vi "LineDraw.vi"(6 "Array":dbl[][](array[numeric]), 8 "Point Y":dbl, 9 "Point X":dbl, 10 "Vehicle Pos Y":dbl, 11 "Vehicle Pos X":dbl) -> (2 "Array 2":dbl[][](array[numeric]))   [LabVIEW 2017]
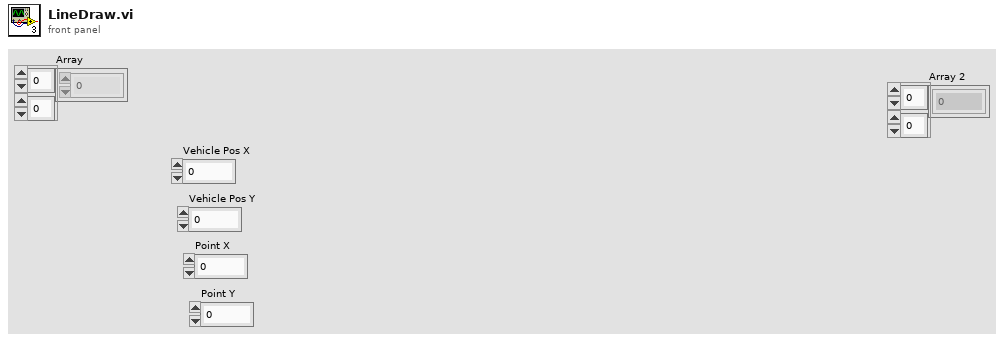
[diagram p1: front panel]
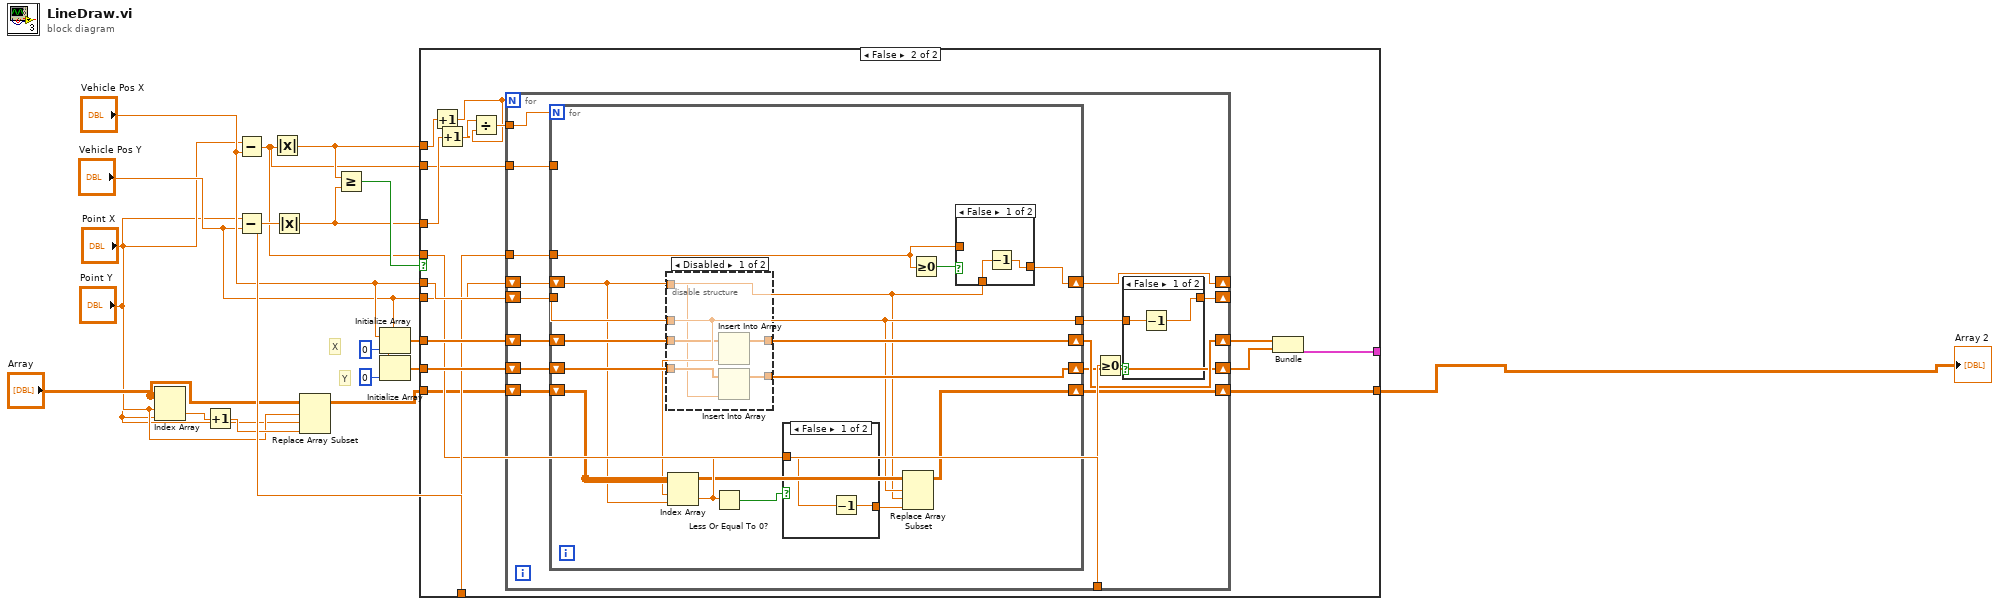
[diagram p0: block diagram]
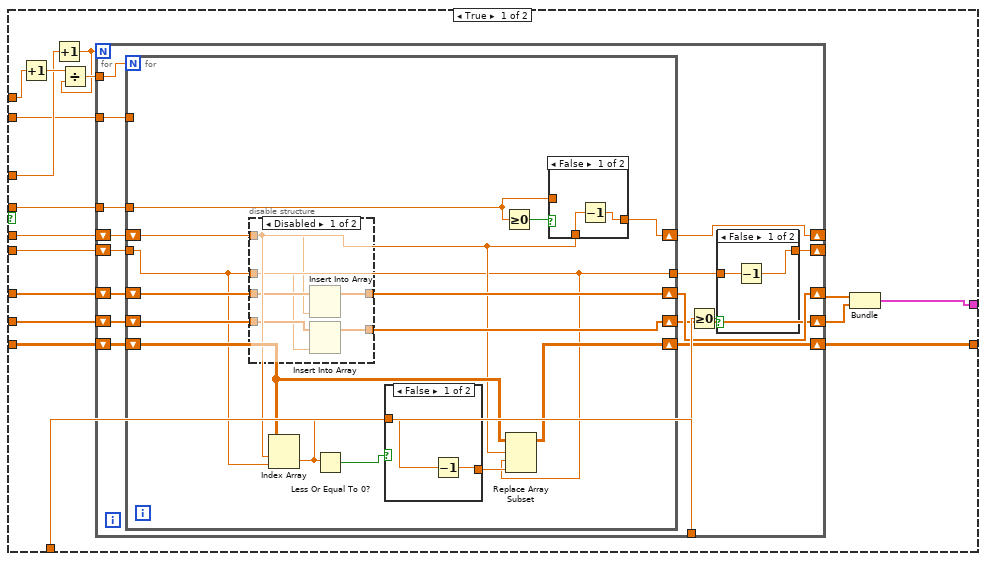
[diagram p2: hidden frame]
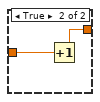
[diagram p3: hidden frame]
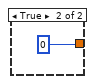
[diagram p5: hidden frame]
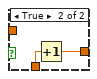
[diagram p6: hidden frame]
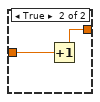
[diagram p7: hidden frame]
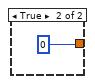
[diagram p9: hidden frame]
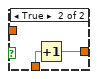
[diagram p10: hidden frame]
diagram:
  # "Y"
  # "X"
  n1 = Index Array(array="Array", index (row)="Point X", index (col)="Point Y") -> (element=w4:dbl)
  n2 = Increment(x=w4) -> (x+1=w3:dbl)
  n3 = Subtract(x="Point X", y="Vehicle Pos X") -> (x-y=w14:dbl)
  n4 = Subtract(x="Point Y", y="Vehicle Pos Y") -> (x-y=w15:dbl)
  n5 = Absolute Value(x=w14) -> (abs(x)=w16:dbl)
  n6 = Absolute Value(x=w15) -> (abs(x)=w17:dbl)
  n7 = Replace Array Subset(array="Array", new element=w3, index (row)="Point X", index (col)="Point Y") -> (w5:dbl[][])
  n8 = Greater Or Equal?(x=w16, y=w17) -> (x >= y?=w18:bool)
  n9 = Initialize Array("Vehicle Pos X", 0 ("dimension size")) -> (w11:dbl[])
  n10 = Initialize Array("Vehicle Pos Y", 0 ("dimension size")) -> (w10:dbl[])
  n11 = case shown="False" w18 {
    tunnel: w5 -> [w20 w84]
    tunnel: w17 -> [w33 w98]
    tunnel: w16 -> [w35 w99]
    tunnel: "Vehicle Pos X" -> [w31 w89]
    tunnel: "Vehicle Pos Y" -> [w30 w88]
    tunnel: w15 -> [w29 w87]
    tunnel: w14 -> [w28 w96]
    tunnel: w14 -> [w27 w86]
    tunnel: w11 -> [w26 w95]
    tunnel: w10 -> [w25 w94]
    tunnel: [w21 w85] -> _
    tunnel: [w19 w83] -> w7
    frame True {
      n12 = Increment(x=w35) -> (x+1=w34:dbl)
      n13 = Increment(x=w33) -> (x+1=w22:dbl)
      n14 = Divide(x=w34, y=w22) -> (x/y=w32:dbl)
      n15 = for {
        N: w22 -> [_]
        tunnel: w32 -> [w51]
        shift-right: [w44] -> _
        shift-left: w30 -> [w46]
        tunnel: w29 -> [w48]
        tunnel: w28 -> [w47]
        tunnel: w27 -> [w45]
        shift-right: [w40] -> w24
        shift-left: w26 -> [w42]
        shift-right: [w39] -> w23
        shift-left: w25 -> [w41]
        shift-right: [w38] -> _
        shift-left: w31 -> [w50]
        shift-right: [w36] -> w19
        shift-left: w20 -> [w37]
        n16 = for {
          N: w51 -> [_]
          shift-right: [w68] -> w38
          shift-left: w50 -> [w57]
          tunnel: w47 -> [_]
          tunnel: w46 -> [w56]
          tunnel: w45 -> [w63]
          tunnel: [w56] -> w43
          shift-right: [w65] -> w40
          shift-left: w42 -> [w67]
          shift-right: [w64] -> w39
          shift-left: w41 -> [w66]
          shift-right: [w58] -> w36
          shift-left: w37 -> [w59]
          n17 = disable-structure shown="Disabled" {
            disable-tunnel: w67 -> [w75 _]
            disable-tunnel: w66 -> [w74 _]
            disable-tunnel: [w73 _] -> w65
            disable-tunnel: [w72 _] -> w64
            disable-tunnel: w57 -> [w71 _]
            disable-tunnel: w56 -> [w70 _]
            frame Disabled {
              n18 = Insert Into Array(array=w75, new element=w71) -> (w73:dbl[])  [unwired: 1 in]
              n19 = Insert Into Array(array=w74, new element=w70) -> (w72:dbl[])  [unwired: 1 in]
            }
            frame Enabled {
            }
          }
          n20 = Index Array(array=w59, index (row)=w57, index (col)=w56) -> (element=w60:dbl)
          n21 = Less Or Equal To 0?(x=w60) -> (x <= 0?=w62:bool)
          n22 = case shown="False" w62 {
            tunnel: [w76 0] -> w61
            tunnel: w60 -> [w77 _]
            frame False {
              n23 = Decrement(x=w77) -> (x-1=w76:dbl)
            }
            frame True {
            }
          }
          n24 = Greater Or Equal To 0?(x=w63) -> (x >= 0?=w69:bool)
          n25 = Replace Array Subset(array=w59, new element=w61, index (row)=w57, index (col)=w56) -> (w58:dbl[][])
          n26 = case shown="False" w69 {
            tunnel: w63 -> [_ _]
            tunnel: w57 -> [w79 w82]
            tunnel: [w80 w81] -> w68
            frame False {
              n27 = Decrement(x=w79) -> (x-1=w80:dbl)
            }
            frame True {
              n28 = Increment(x=w82) -> (x+1=w81:dbl)
            }
          }
        }
        n29 = Greater Or Equal To 0?(x=w48) -> (x >= 0?=w49:bool)
        n30 = case shown="False" w49 {
          tunnel: [w53 w55] -> w44
          tunnel: w43 -> [w52 w54]
          frame False {
            n31 = Decrement(x=w52) -> (x-1=w53:dbl)
          }
          frame True {
            n32 = Increment(x=w54) -> (x+1=w55:dbl)
          }
        }
      }
      n33 = Bundle(w24, w23) -> (w21:cluster{dbl[], dbl[]})  [unwired: 1 in]
    }
    frame False {
      n34 = Increment(x=w99) -> (x+1=w91:dbl)
      n35 = Increment(x=w98) -> (x+1=w90:dbl)
      n36 = Divide(x=w90, y=w91) -> (x/y=w97:dbl)
      n37 = for {
        N: w91 -> [_]
        tunnel: w97 -> [w102]
        shift-right: [w109] -> _
        shift-left: w89 -> [w111]
        tunnel: w86 -> [w113]
        tunnel: w96 -> [w112]
        tunnel: w87 -> [w110]
        shift-right: [w105] -> w93
        shift-left: w95 -> [w107]
        shift-right: [w104] -> w92
        shift-left: w94 -> [w106]
        shift-right: [w103] -> _
        shift-left: w88 -> [w115]
        shift-right: [w100] -> w83
        shift-left: w84 -> [w101]
        n38 = for {
          N: w102 -> [_]
          shift-right: [w132] -> w103
          shift-left: w115 -> [w122]
          tunnel: w112 -> [_]
          tunnel: w111 -> [w123]
          tunnel: w110 -> [w127]
          tunnel: [w123] -> w108
          shift-right: [w129] -> w105
          shift-left: w107 -> [w131]
          shift-right: [w128] -> w104
          shift-left: w106 -> [w130]
          shift-right: [w120] -> w100
          shift-left: w101 -> [w124]
          n39 = disable-structure shown="Disabled" {
            disable-tunnel: w131 -> [w139 _]
            disable-tunnel: w130 -> [w138 _]
            disable-tunnel: [w137 _] -> w129
            disable-tunnel: [w136 _] -> w128
            disable-tunnel: w123 -> [w135 _]
            disable-tunnel: w122 -> [w134 _]
            frame Disabled {
              n40 = Insert Into Array(array=w139, new element=w135) -> (w137:dbl[])  [unwired: 1 in]
              n41 = Insert Into Array(array=w138, new element=w134) -> (w136:dbl[])  [unwired: 1 in]
            }
            frame Enabled {
            }
          }
          n42 = Index Array(array=w124, index (row)=w123, index (col)=w122) -> (element=w125:dbl)
          n43 = Less Or Equal To 0?(x=w125) -> (x <= 0?=w126:bool)
          n44 = case shown="False" w126 {
            tunnel: [w140 0] -> w121
            tunnel: w125 -> [w141 _]
            frame False {
              n45 = Decrement(x=w141) -> (x-1=w140:dbl)
            }
            frame True {
            }
          }
          n46 = Replace Array Subset(array=w124, new element=w121, index (row)=w123, index (col)=w122) -> (w120:dbl[][])
          n47 = Greater Or Equal To 0?(x=w127) -> (x >= 0?=w133:bool)
          n48 = case shown="False" w133 {
            tunnel: w127 -> [_ _]
            tunnel: w122 -> [w143 w146]
            tunnel: [w144 w145] -> w132
            frame False {
              n49 = Decrement(x=w143) -> (x-1=w144:dbl)
            }
            frame True {
              n50 = Increment(x=w146) -> (x+1=w145:dbl)
            }
          }
        }
        n51 = Greater Or Equal To 0?(x=w113) -> (x >= 0?=w114:bool)
        n52 = case shown="False" w114 {
          tunnel: [w117 w119] -> w109
          tunnel: w108 -> [w116 w118]
          frame False {
            n53 = Decrement(x=w116) -> (x-1=w117:dbl)
          }
          frame True {
            n54 = Increment(x=w118) -> (x+1=w119:dbl)
          }
        }
      }
      n55 = Bundle(w93, w92) -> (w85:cluster{dbl[], dbl[]})  [unwired: 1 in]
    }
  }
  "Array 2" <- w7
